vi "Format Fiducial Slot.vi"(4 "Slot":i32, 6 "Chuck":i32, 7 "Part Type":T1, 8 "error in":errorcluster, 9 "Fiducials":T2[](array[typedef]), 10 "Location/Orientation":T6, 11 "Console Log in":refnum<class "Console Log.lvclass">) -> (0 "error out":errorcluster, 2 "Array":string[](array[string]), 3 "Console Log out":refnum<class "Console Log.lvclass">)   [LabVIEW 2011, in "Console Log.lvclass"]
uses:
  Console Log.lvclass
  Shared Components/Utils/Type Definitions/Position_Orientation.ctl
  Shared Components/Vec3d Class/Vec3d Class.lvclass
  Shared Components/Orient3d Class/Orient3d Class.lvclass
  Shared Components/Utils/Type Definitions/Fiducial Image.ctl
  Shared Components/Utils/Type Definitions/Physical Image.ctl
  <vilib>/vision/Image Controls.llb/IMAQ Image.ctl
  Shared Components/Utils/Type Definitions/Fiducial with Source.ctl
  Shared Components/Config Manager Class/Type Definitions/Part Type.ctl
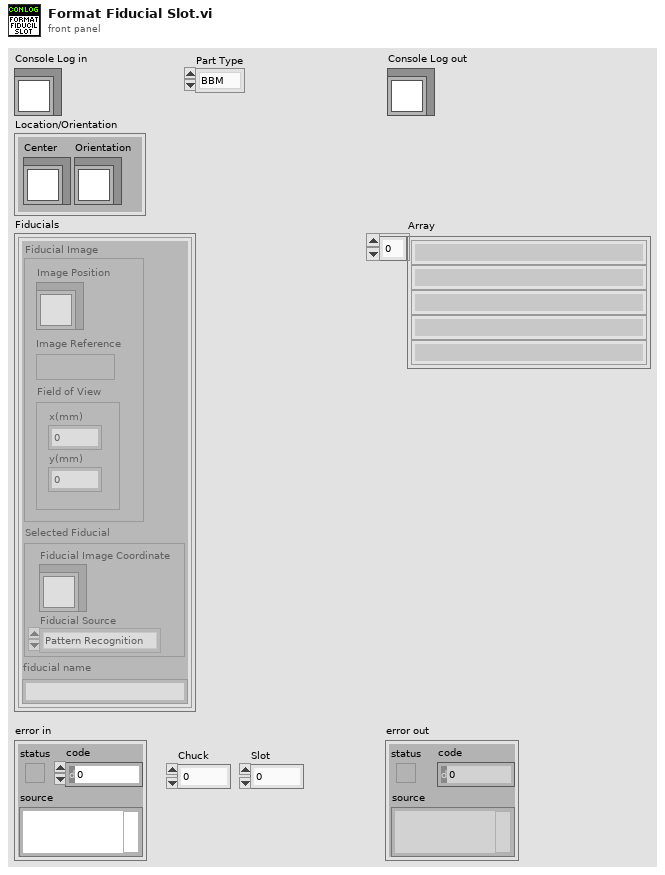
[diagram p1: front panel]
types:
  T1 = typedef "Part Type.ctl" = enum16{"BBM", "HDI", "BARE HDI", "GLUERESERVOIR", "STAMP_1", "STAMP_2", "STAMP_3", "STAMP_4", "STAMP_5", "WEIGHT_1", "WEIGHT_2", "WEIGHT_3", "WEIGHT_4", "WEIGHT_5", "WEIGHT_6", "WEIGHT_7", "WEIGHT_8", "PICKER_TOOL", "GRABER_TOOL"}
  T2 = typedef "Fiducial Image.ctl" = cluster{"Fiducial Image":T3, "Selected Fiducial":T5, "fiducial name":string}
  T3 = typedef "Physical Image.ctl" = cluster{"Image Position":refnum<class "Vec3d Class.lvclass">, "Image Reference":T4, "Field of View":cluster{"x(mm)":dbl, "y(mm)":dbl}}
  T4 = typedef "IMAQ Image.ctl" = refnum<image>
  T5 = typedef "Fiducial with Source.ctl" = cluster{"Fiducial Image Coordinate":refnum<class "Vec3d Class.lvclass">, "Fiducial Source":enum16{"Pattern Recognition", "User", "Error", "Default"}}
  T6 = typedef "Position_Orientation.ctl" = cluster{"Center":refnum<class "Vec3d Class.lvclass">, "Orientation":refnum<class "Orient3d Class.lvclass">}
  T7 = enum16{"Pattern Recognition", "User", "Error", "Default"}
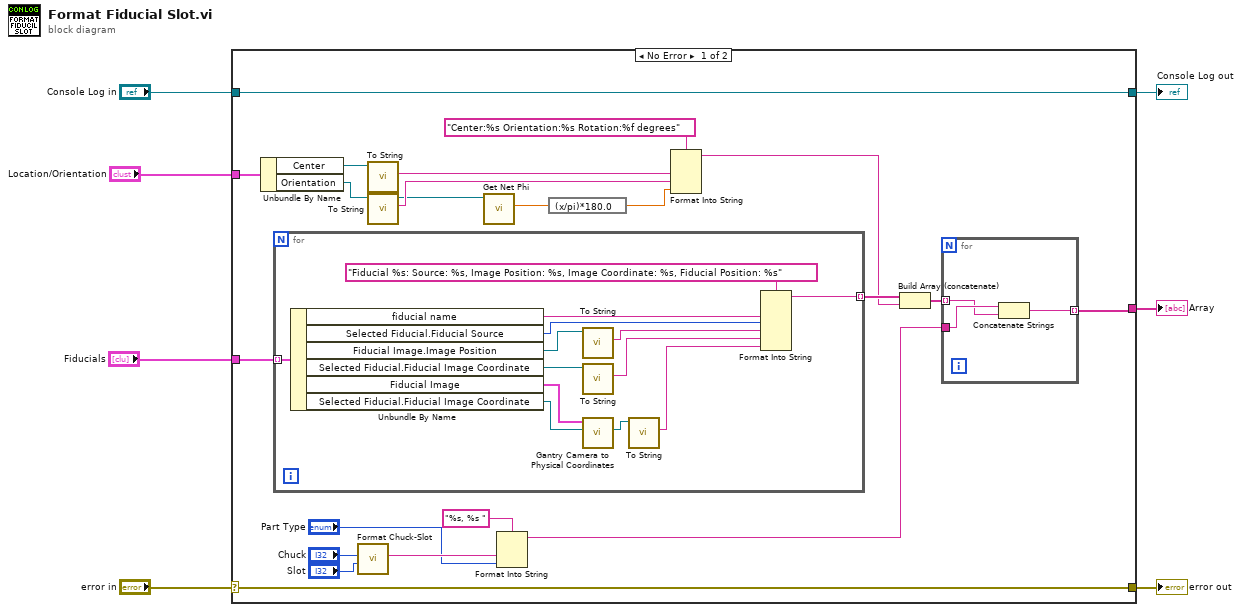
[diagram p0: block diagram]
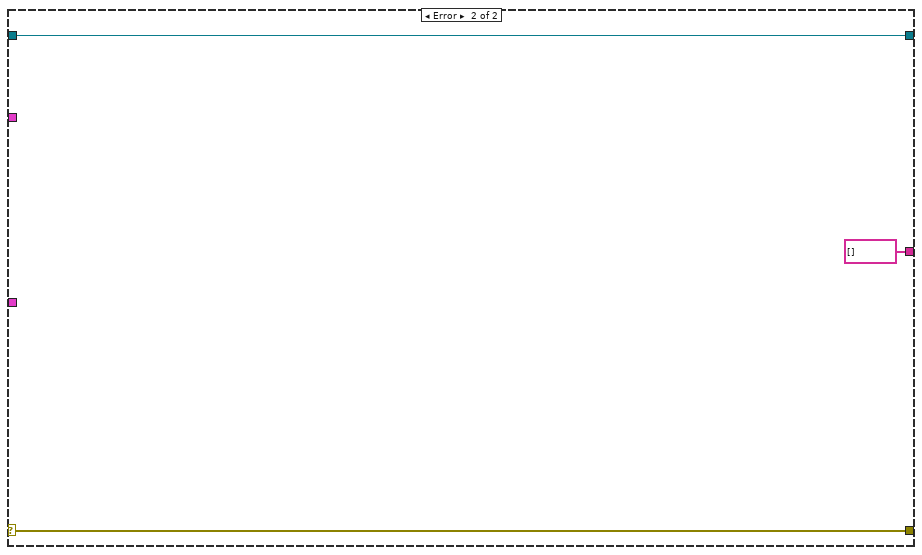
[diagram p2: hidden frame]
diagram:
  n1 = case shown="No Error" "error in" {
    selector: "error in" -> [w28 w48]
    tunnel: [w28 w48] -> w6
    tunnel: [w29 w47] -> w4
    tunnel: "Console Log in" -> [w29 w47]
    tunnel: "Location/Orientation" -> [w27 _]
    tunnel: "Fiducials" -> [w20 _]
    tunnel: [w12 string[] []] -> w1
    frame No Error {
      n2 = Unbundle By Name(w27) -> ("Center"=w26:refnum<class "Vec3d Class.lvclass">, "Orientation"=w25:refnum<class "Orient3d Class.lvclass">)
      n3 = for {
        tunnel: w20 -> [w45] mode=indexing
        tunnel: [w33] -> w16 mode=indexing
        n4 = Unbundle By Name(w45) -> ("fiducial name"=w43:string, "Selected Fiducial.Fiducial Source"=w42:T7, "Fiducial Image.Image Position"=w41:refnum<class "Vec3d Class.lvclass">, "Selected Fiducial.Fiducial Image Coordinate"=w39:refnum<class "Vec3d Class.lvclass">, "Fiducial Image"=w37:T3, "Selected Fiducial.Fiducial Image Coordinate"=w36:refnum<class "Vec3d Class.lvclass">)
        n5 = call "To String.vi"("Vec3d in"=w41) -> ("Vec3d String"=w40:string)  [unwired: 8 in, 2 out]
        n6 = call "To String.vi"("Vec3d in"=w39) -> ("Vec3d String"=w38:string)  [unwired: 8 in, 2 out]
        n7 = call "Gantry Camera to Physical Coordinates.vi"("Image Coordinate"=w36, "Physical Image"=w37) -> ("Global Coordinate"=w35:refnum<class "Vec3d Class.lvclass">)  [unwired: 7 in, 2 out]
        n8 = call "To String.vi"("Vec3d in"=w35) -> ("Vec3d String"=w34:string)  [unwired: 8 in, 2 out]
        n9 = Format Into String(format string="Fiducial %s: Source: %s, Image Position: %s, Image Coordinate: %s, Fiducial Position: %s", w43, w42, w40, w38, w34) -> (resulting string=w33:string)  [unwired: 2 in, 1 out]
      }
      n10 = call "Format Chuck-Slot.vi"("Slot"="Slot", "Chuck"="Chuck") -> ("Formatted Chuck/Slot"=w18:string)  [unwired: 7 in, 2 out]
      n11 = call "To String.vi"("Vec3d in"=w26) -> ("Vec3d String"=w21:string)  [unwired: 8 in, 2 out]
      n12 = call "To String.vi"("Orient3d in"=w25) -> ("Orient3d String"=w11:string, "Orient3d out"=w10:refnum<class "Orient3d Class.lvclass">)  [unwired: 8 in, 1 out]
      n13 = call "Get Net Phi.vi"("Orient3d"=w10) -> ("phi(rad)"=w9:dbl)  [unwired: 8 in, 2 out]
      n14 = Format Into String(format string="%s, %s ", w18, "Part Type") -> (resulting string=w13:string)  [unwired: 2 in, 1 out]
      n15 = expression code="(x/pi)*180.0" ("radians to degrees")(w9) -> (w8:dbl)
      n16 = Format Into String(format string="Center:%s Orientation:%s Rotation:%f degrees", w21, w11, w8) -> (resulting string=w15:string)  [unwired: 2 in, 1 out]
      n17 = Build Array (concatenate)(w16, w15) -> (w14:string[])
      n18 = for {
        tunnel: w14 -> [w31] mode=indexing
        tunnel: w13 -> [w32]
        tunnel: [w30] -> w12 mode=indexing
        n19 = Concatenate Strings(w32, w31) -> (w30:string)
      }
    }
    frame Error {
    }
  }
  "error out" <- w6
  "Console Log out" <- w4
  "Array" <- w1
